vi "Signal analysis.vi"() -> ()   [LabVIEW 2014]
uses:
  <vilib>/Utility/file.llb/Write To Spreadsheet File (DBL).vi
panel:
  in  "Write Raw  signal temperature":bool
  in  "Write Raw signal pressure":bool
  in  "stop":bool
  in  "Write Signal Statistics":bool
  out "Waveform Graph 3":dynamicdata(graph)
  out "Waveform Graph 2":dynamicdata(graph)
  in  "Filter 2":bool
  in  "Filter":bool
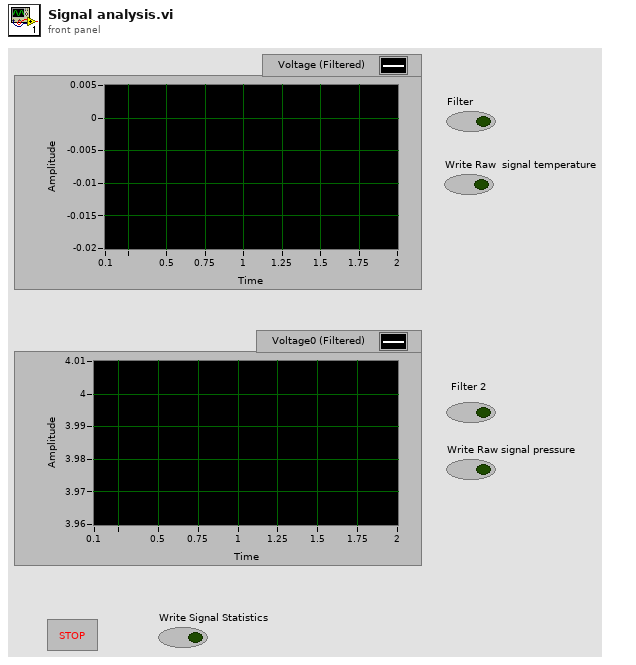
[diagram p1: front panel]
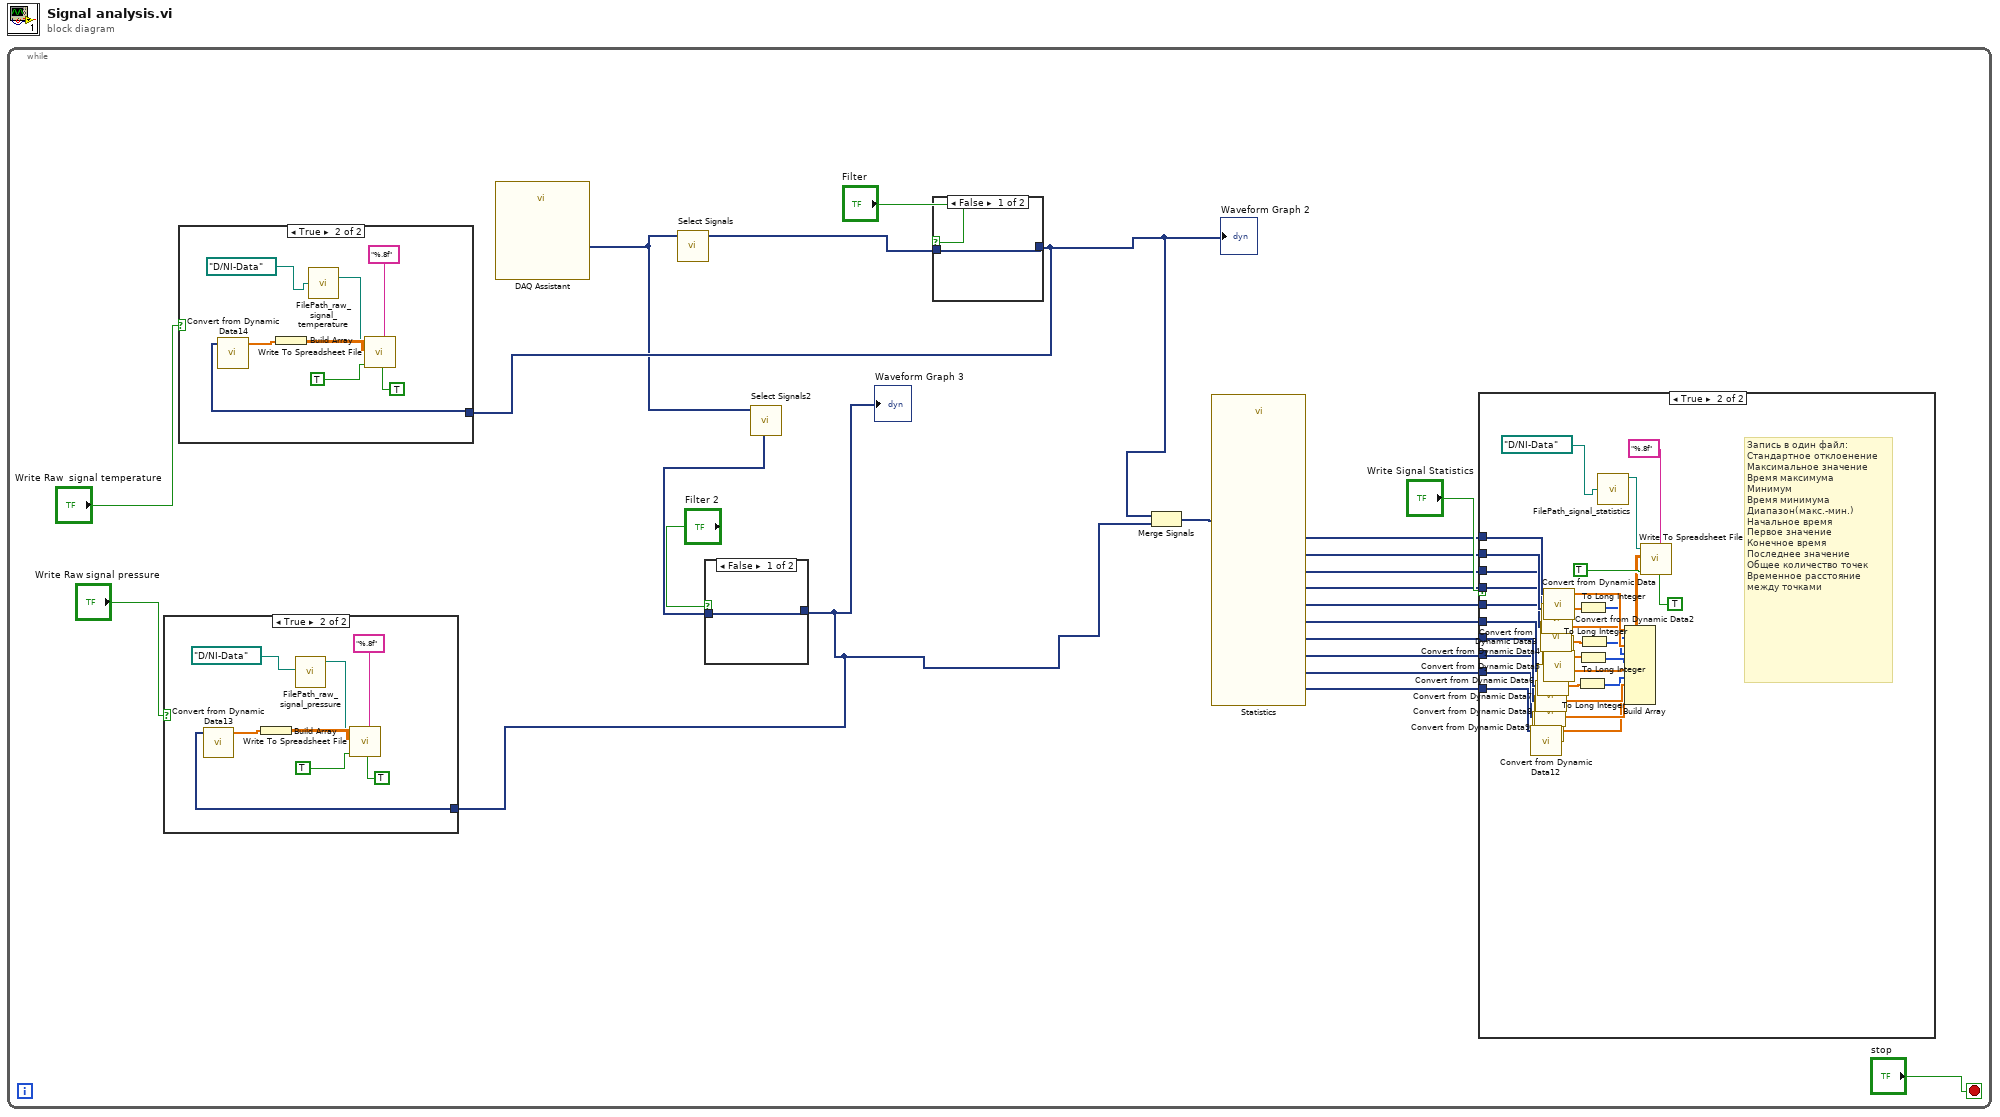
[diagram p0: block diagram]
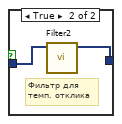
[diagram p5: hidden frame]
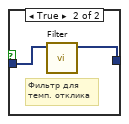
[diagram p6: hidden frame]
diagram:
  n1 = while {
    stop <- "stop" stop-if-true
    n2 = call "DAQ Assistant"() -> ("data"=w2:dynamicdata)  [unwired: 2 in, 9 out]
    n3 = call "Select Signals"("Signals"=w2) -> ("Signal Out"=w1:dynamicdata)  [unwired: 1 in, 9 out]
    n4 = call "Select Signals2"("Signals"=w2) -> ("Signal Out"=w21:dynamicdata)  [unwired: 1 in, 9 out]
    n5 = case shown="False" "Filter 2" {
      tunnel: w21 -> [w69 w71]
      tunnel: [w69 w70] -> w3
      frame False {
      }
      frame True {
        # "Фильтр для\nтемп. отклика"
        n6 = call "Filter2"("Signal"=w71) -> ("Filtered Signal"=w70:dynamicdata)  [unwired: 2 in, 8 out]
      }
    }
    "Waveform Graph 3" <- w3
    n7 = case shown="True" "Write Raw signal pressure" {
      tunnel: w3 -> [_ w33]
      frame False {
      }
      frame True {
        n8 = call "Convert from Dynamic Data13"("Dynamic Data Type"=w33) -> ("Array"=w34:dbl[])  [unwired: 3 in]
        n9 = Build Array(w34) -> (w35:dbl[][])
        n10 = call "FilePath_raw_signal_pressure.vi"("base folder path"=path "D:/NI-Data") -> ("Raw_data_path"=w31:path)  [unwired: 3 in]
        n11 = call-poly <vilib>:"Write To Spreadsheet File.vi"("transpose? (no:F)"=TRUE, "format (%.3f)"="%.8f", "append to file? (new file:F)"=TRUE, "2D data"=w35, "file path (dialog if empty)"=w31) -> ()  [unwired: 1 in, 3 out]
      }
    }
    n12 = case shown="False" "Filter" {
      tunnel: w1 -> [w72 w74]
      tunnel: [w72 w73] -> w4
      frame False {
      }
      frame True {
        # "Фильтр для\nтемп. отклика"
        n13 = call "Filter"("Signal"=w74) -> ("Filtered Signal"=w73:dynamicdata)  [unwired: 2 in, 8 out]
      }
    }
    "Waveform Graph 2" <- w4
    n14 = case shown="True" "Write Raw  signal temperature" {
      tunnel: w4 -> [_ w25]
      frame False {
      }
      frame True {
        n15 = call "Convert from Dynamic Data14"("Dynamic Data Type"=w25) -> ("Array"=w26:dbl[])  [unwired: 3 in]
        n16 = Build Array(w26) -> (w27:dbl[][])
        n17 = call "FilePath_raw_signal_temperature.vi"("base folder path"=path "D:/NI-Data") -> ("Raw_data_path"=w24:path)  [unwired: 3 in]
        n18 = call-poly <vilib>:"Write To Spreadsheet File.vi"("transpose? (no:F)"=TRUE, "format (%.3f)"="%.8f", "append to file? (new file:F)"=TRUE, "2D data"=w27, "file path (dialog if empty)"=w24) -> ()  [unwired: 1 in, 3 out]
      }
    }
    n19 = Merge Signals(w4, w3) -> (w7:dynamicdata)
    n20 = call "Statistics"("Signals"=w7) -> ("Total Samples"=w9:dynamicdata, "Time Delta"=w8:dynamicdata, "Last Value"=w10:dynamicdata, "Last Time"=w11:dynamicdata, "First Value"=w12:dynamicdata, "First Time"=w13:dynamicdata, "Time of Minimum"=w14:dynamicdata, "Minimum"=w15:dynamicdata, "Time of Maximum"=w16:dynamicdata, "Maximum"=w17:dynamicdata)  [unwired: 16 in, 1 out]
    n21 = case shown="True" "Write Signal Statistics" {
      tunnel: w17 -> [_ w62]
      tunnel: w16 -> [_ w61]
      tunnel: w15 -> [_ w60]
      tunnel: w14 -> [_ w59]
      tunnel: w13 -> [_ w58]
      tunnel: w12 -> [_ w57]
      tunnel: w11 -> [_ w56]
      tunnel: w10 -> [_ w55]
      tunnel: w9 -> [_ w54]
      tunnel: w8 -> [_ w53]
      frame False {
      }
      frame True {
        # "Запись в один файл:\nСтандартное отклоенение\nМаксимальное значение\nВремя максимума\nМинимум\nВремя минимума\nДиапазон(макс.-мин.)\nНачальное время\nПервое значение\nКонечное время\nПоследнее значение\nОбщее количество точек\nВременное расстояние между точками"
        n22 = call "Convert from Dynamic Data12"("Dynamic Data Type"=w53) -> ("Array"=w48:dbl[])  [unwired: 3 in]
        n23 = call "Convert from Dynamic Data9"("Dynamic Data Type"=w54) -> ("Array"=w49:dbl[])  [unwired: 3 in]
        n24 = call "Convert from Dynamic Data8"("Dynamic Data Type"=w55) -> ("Array"=w50:dbl[])  [unwired: 3 in]
        n25 = call "Convert from Dynamic Data7"("Dynamic Data Type"=w56) -> ("Array"=w40:dbl[])  [unwired: 3 in]
        n26 = call "Convert from Dynamic Data6"("Dynamic Data Type"=w57) -> ("Array"=w41:dbl[])  [unwired: 3 in]
        n27 = call "Convert from Dynamic Data3"("Dynamic Data Type"=w60) -> ("Array"=w51:dbl[])  [unwired: 3 in]
        n28 = call "Convert from Dynamic Data2"("Dynamic Data Type"=w61) -> ("Array"=w45:dbl[])  [unwired: 3 in]
        n29 = call "Convert from Dynamic Data4"("Dynamic Data Type"=w59) -> ("Array"=w47:dbl[])  [unwired: 3 in]
        n30 = call "Convert from Dynamic Data"("Dynamic Data Type"=w62) -> ("Array"=w52:dbl[])  [unwired: 3 in]
        n31 = call "Convert from Dynamic Data5"("Dynamic Data Type"=w58) -> ("Array"=w43:dbl[])  [unwired: 3 in]
        n32 = To Long Integer(number=w40) -> (32bit integer=w39:i32[])
        n33 = To Long Integer(number=w45) -> (32bit integer=w44:i32[])
        n34 = To Long Integer(number=w43) -> (32bit integer=w42:i32[])
        n35 = To Long Integer(number=w47) -> (32bit integer=w46:i32[])
        n36 = call "FilePath_signal_statistics.vi"("base folder path"=path "D:/NI-Data") -> ("Signal_path"=w63:path)  [unwired: 3 in]
        n37 = Build Array(w52, w44, w51, w46, w42, w41, w39, w50, w49, w48) -> (w65:dbl[][])
        n38 = call-poly <vilib>:"Write To Spreadsheet File.vi"("transpose? (no:F)"=TRUE, "format (%.3f)"="%.8f", "append to file? (new file:F)"=TRUE, "2D data"=w65, "file path (dialog if empty)"=w63) -> ()  [unwired: 1 in, 3 out]
      }
    }
  }
